vi "Imagen a angulo.vi"(8 "error in (no error)":errorcluster, 9 "Imagen destino (in)":T1, 10 "Imagen original":T1, 11 "Sesion de camara (in)":T2) -> (0 "error out":errorcluster, 1 "Imagen destino (out)":T1, 2 "Variable de proceso":dbl, 3 "Sesion de camara (out)":T2)   [LabVIEW 2020]
uses:
  <vilib>/vision/Image Controls.llb/IMAQ Image.ctl
  <vilib>/userdefined/High Color/IMAQdx.ctl
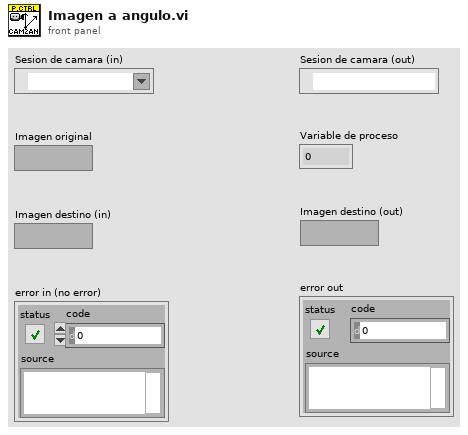
[diagram p1: front panel]
types:
  T1 = typedef "IMAQ Image.ctl" = refnum<image>
  T2 = typedef "IMAQdx.ctl" = refnum<k21>
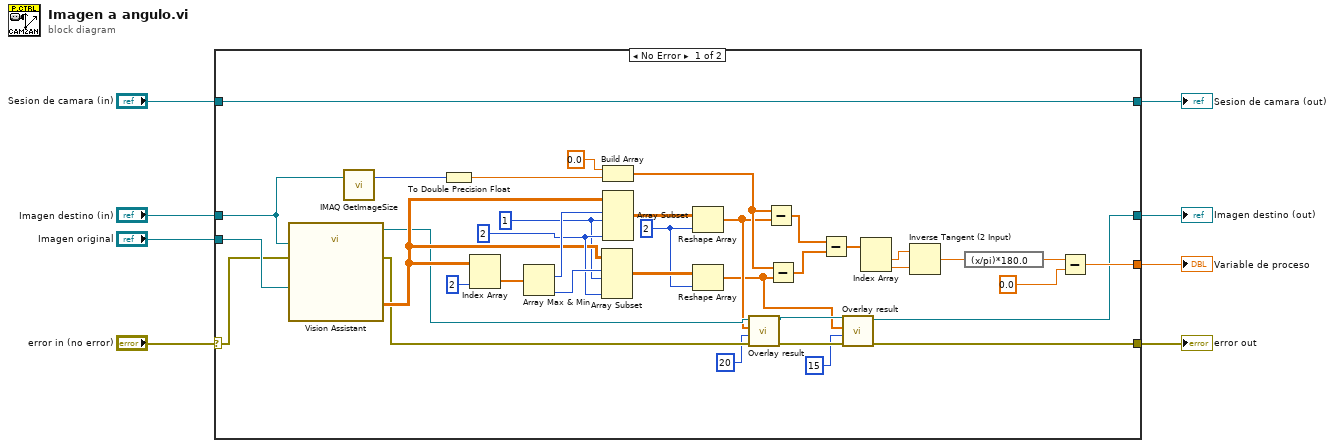
[diagram p0: block diagram]
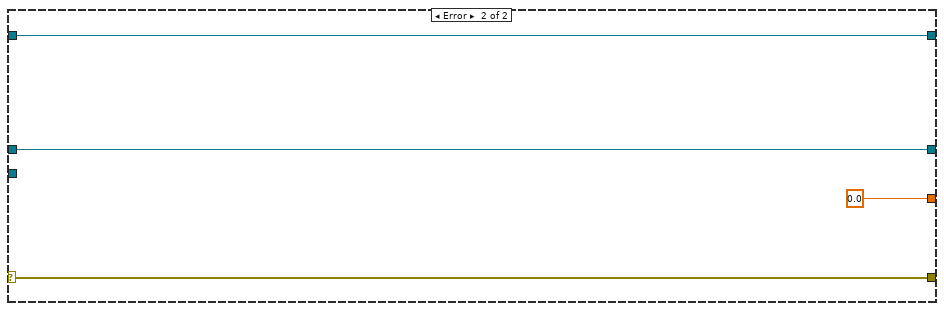
[diagram p2: hidden frame]
diagram:
  n1 = case shown="No Error" "error in (no error)" {
    selector: "error in (no error)" -> [w43 w49]
    tunnel: [w12 w48] -> w2
    tunnel: "Imagen destino (in)" -> [w33 w48]
    tunnel: "Imagen original" -> [w45 _]
    tunnel: [w44 w46] -> w6
    tunnel: "Sesion de camara (in)" -> [w44 w46]
    tunnel: [w11 w49] -> w4
    tunnel: [w21 0.0] -> w1
    frame No Error {
      w34 = 2 ("dimension size")
      w36 = 1 ("length")
      w38 = 2 ("length")
      n2 = call "Vision Assistant"("Image In"=w45, "Image Dst"=w33, "error in"=w43) -> ("Image Out"=w19:T1, "Particle Measurements (Pixels) (Particle Analysis 2)"=w37:dbl[][], "error out"=w16:errorcluster)  [unwired: 22 in]
      n3 = call "IMAQ GetImageSize"("Image"=w33) -> ("Y Resolution"=w32:i32)  [unwired: 3 in, 2 out]
      n4 = To Double Precision Float(number=w32) -> (double precision float=w30:dbl)
      n5 = Index Array(array=w37, index (col)=2 ("disabled index (col)")) -> (element=w41:dbl[])  [unwired: 1 in]
      n6 = Array Max & Min(array=w41) -> (max index (indices)=w40:i32, min index (indices)=w39:i32)  [unwired: 2 out]
      n7 = Array Subset(array=w37, index (row)=w39, length (row)=w36, length (col)=w38) -> (w35:dbl[][])  [unwired: 1 in]
      n8 = Build Array(0.0 ("element"), w30) -> (w20:dbl[])
      n9 = Array Subset(array=w37, index (row)=w40, length (row)=w36, length (col)=w38) -> (w18:dbl[][])  [unwired: 1 in]
      n10 = Reshape Array(w18, w34) -> (w17:dbl[])
      n11 = Reshape Array(w35, w34) -> (w10:dbl[])
      n12 = call "Overlay result.vi"("error in (no error)"=w16, "Size"=20, "Array"=w17, "Image in"=w19) -> ("error out"=w14:errorcluster, "Image out"=w13:T1)  [unwired: 6 in]
      n13 = Subtract(x=w20, y=w17) -> (x-y=w29:dbl[])
      n14 = Subtract(x=w20, y=w10) -> (x-y=w28:dbl[])
      n15 = Subtract(x=w29, y=w28) -> (x-y=w27:dbl[])
      n16 = call "Overlay result.vi"("error in (no error)"=w14, "Size"=15, "Array"=w10, "Image in"=w13) -> ("error out"=w11:errorcluster, "Image out"=w12:T1)  [unwired: 6 in]
      n17 = Index Array(array=w27) -> (element #1=w26:dbl, element #2=w25:dbl)  [unwired: 2 in]
      n18 = Inverse Tangent (2 Input)(1:w25, 2:w26) -> (0:w24:dbl)
      n19 = expression code="(x/pi)*180.0" ("radians to degrees")(w24) -> (w23:dbl)
      n20 = Subtract(x=w23, y=0.0) -> (x-y=w21:dbl)
    }
    frame Error {
    }
  }
  "Sesion de camara (out)" <- w6
  "error out" <- w4
  "Imagen destino (out)" <- w2
  "Variable de proceso" <- w1
